vi "Write Initialised_.vi"(8 "error in (no error)":errorcluster, 10 "Initialised?":bool, 11 "Singleton in":refnum<class "Singleton.lvclass">) -> (0 "error out":errorcluster, 3 "Singleton out":refnum<class "Singleton.lvclass">)   [LabVIEW 2020, in "Singleton.lvlib" / "Singleton.lvclass"]
uses:
  Singleton.lvclass
  Singleton.lvclass/Singleton.ctl
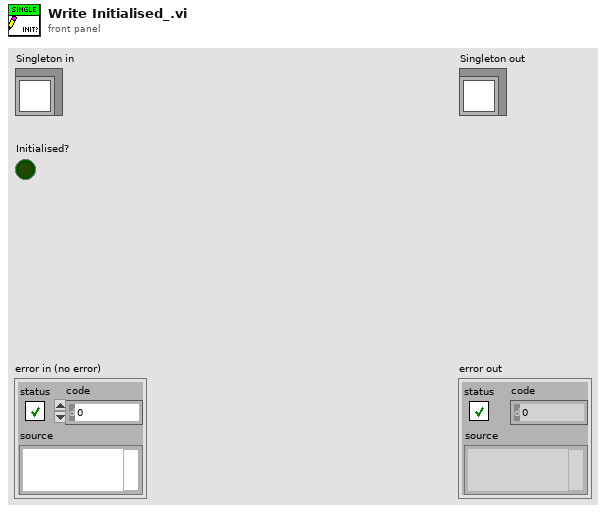
[diagram p1: front panel]
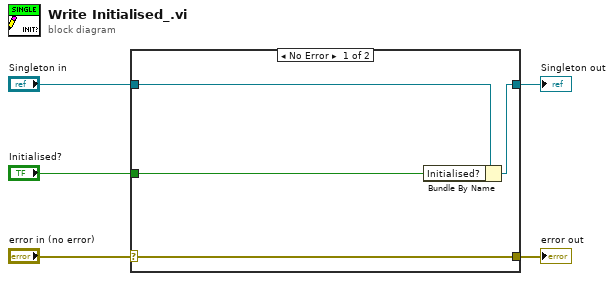
[diagram p0: block diagram]
diagram:
  n1 = case shown="No Error" "error in (no error)" {
    selector: "error in (no error)" -> [w9 w10]
    tunnel: [w9 w10] -> w4
    tunnel: [w7 w11] -> w2
    tunnel: "Singleton in" -> [w8 w11]
    tunnel: "Initialised?" -> [w6 _]
    frame No Error {
      n2 = Bundle By Name(cluster=w8, "Initialised?"=w6) -> (w7:refnum<class "Singleton.lvclass">)
    }
    frame Error {
    }
  }
  "error out" <- w4
  "Singleton out" <- w2
